vi "Read Element of AM Enabled.vi"(8 "error in (no error)":errorcluster, 10 "index":i32, 11 "CS++FgenChannelData in":refnum<class "CS++FgenChannelData.lvclass">) -> (0 "error out":errorcluster, 2 "AM enabled (True)":bool=TRUE, 3 "CS++FgenChannelData out":refnum<class "CS++FgenChannelData.lvclass">)   [LabVIEW 2015, in "CS++FgenGui.lvlib" / "CS++FgenChannelData.lvclass"]
uses:
  CS++FgenChannelData.lvclass
  CS++FgenChannelData.lvclass/CS++FgenChannelData.ctl
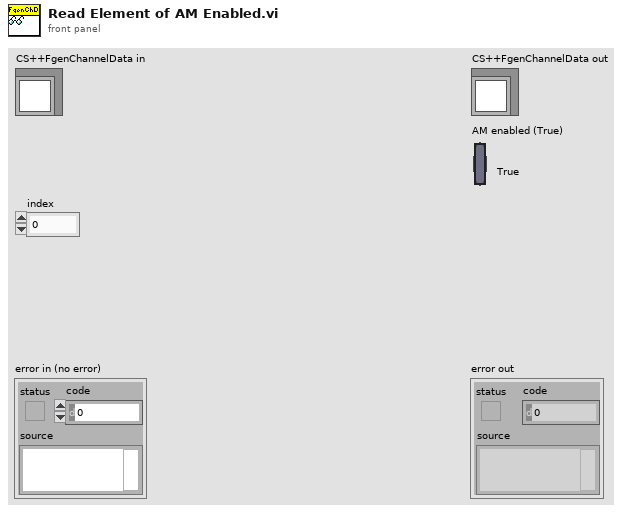
[diagram p1: front panel]
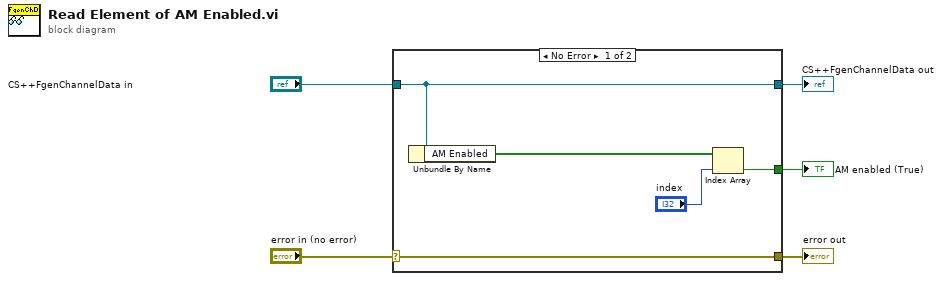
[diagram p0: block diagram]
diagram:
  n1 = case shown="No Error" "error in (no error)" {
    selector: "error in (no error)" -> [w10 w11]
    tunnel: [w10 w11] -> w4
    tunnel: [w9 w12] -> w2
    tunnel: "CS++FgenChannelData in" -> [w9 w12]
    tunnel: [w6 _] -> w1
    frame No Error {
      n2 = Unbundle By Name(w9) -> ("AM Enabled"=w8:bool[])
      n3 = Index Array(array=w8, index="index") -> (element=w6:bool)
    }
    frame Error {
    }
  }
  "error out" <- w4
  "CS++FgenChannelData out" <- w2
  "AM enabled (True)" <- w1
